vi "Talon Velocity Control.vi"(0 "CAN Talon SRX Ref":T1={"DeviceStatus"={"status"=FALSE, "code"=0, "source"=""}, "Type"=enum."PWM", "PWM"={"PWM Channel"=enum."PWM 1", "DeadBand"={"Name"="", "maxPositivePwm"=0, "minPositivePwm"=0, "centerPwm"=0, "maxNegativePwm"=0, "minNegativePwm"=0, "angularRange"=0}}, "CAN"={"Device Number"=0, "Control Mode"=enum."Percent VBus", "Semaphore"=refnum, "Max Vout"=12.0, "TalonSRX Control Mode"=enum."Percent VBus"}, "Invert"=FALSE}, 5 "PercentVoltage":dbl, 7 "Run to Speed?":bool, 9 "TargetSpeedRPM":dbl, 11 "error in (no error)":errorcluster) -> (4 "CAN Talon SRX Ref":T1={"DeviceStatus"={"status"=FALSE, "code"=0, "source"=""}, "Type"=enum."PWM", "PWM"={"PWM Channel"=enum."Invalid", "DeadBand"={"Name"="", "maxPositivePwm"=0, "minPositivePwm"=0, "centerPwm"=0, "maxNegativePwm"=0, "minNegativePwm"=0, "angularRange"=0}}, "CAN"={"Device Number"=0, "Control Mode"=enum."Percent VBus", "Semaphore"=refnum, "Max Vout"=12.0, "TalonSRX Control Mode"=enum."Percent VBus"}, "Invert"=FALSE}, 6 "Control Mode":T7, 10 "Motor Set":dbl, 15 "error out":errorcluster)   [LabVIEW 2015]
uses:
  <vilib>/Rock Robotics/WPI/MotorControl/WPI_MotorControlDeviceRef.ctl
  <vilib>/Rock Robotics/WPI/MotorControl/WPI_MotorControlType.ctl
  <vilib>/Rock Robotics/SystemInterfaces/DIO/FPGA_DIOPWMChannel.ctl
  <vilib>/Rock Robotics/WPI/PWM/WPI_PWMDeadband.ctl
  <vilib>/Rock Robotics/WPI/CAN/Jaguar/SubVIs/WPI_CANJaguar_ControlMode.ctl
  <vilib>/Rock Robotics/WPI/CAN/TalonSRX/WPI_CANTalonSRX_APIControlMode.ctl
  <vilib>/Rock Robotics/WPI/CAN/TalonSRX/WPI_CANTalonSRX_APIFeedbackSelect.ctl
panel:
  in  "PID stuff":T8
  out "SensorPosRotations":dbl
  out "Motor output Plot":cluster{"Applied Throttle":dbl}(graph)
  out "Target RPM":dbl
  out "SensorRPM Velocity RPM":dbl
  out "Applied Output":dbl
  out "Speed Closed Loop Plots":cluster{dbl, "Sensor Velocity":dbl}(graph)
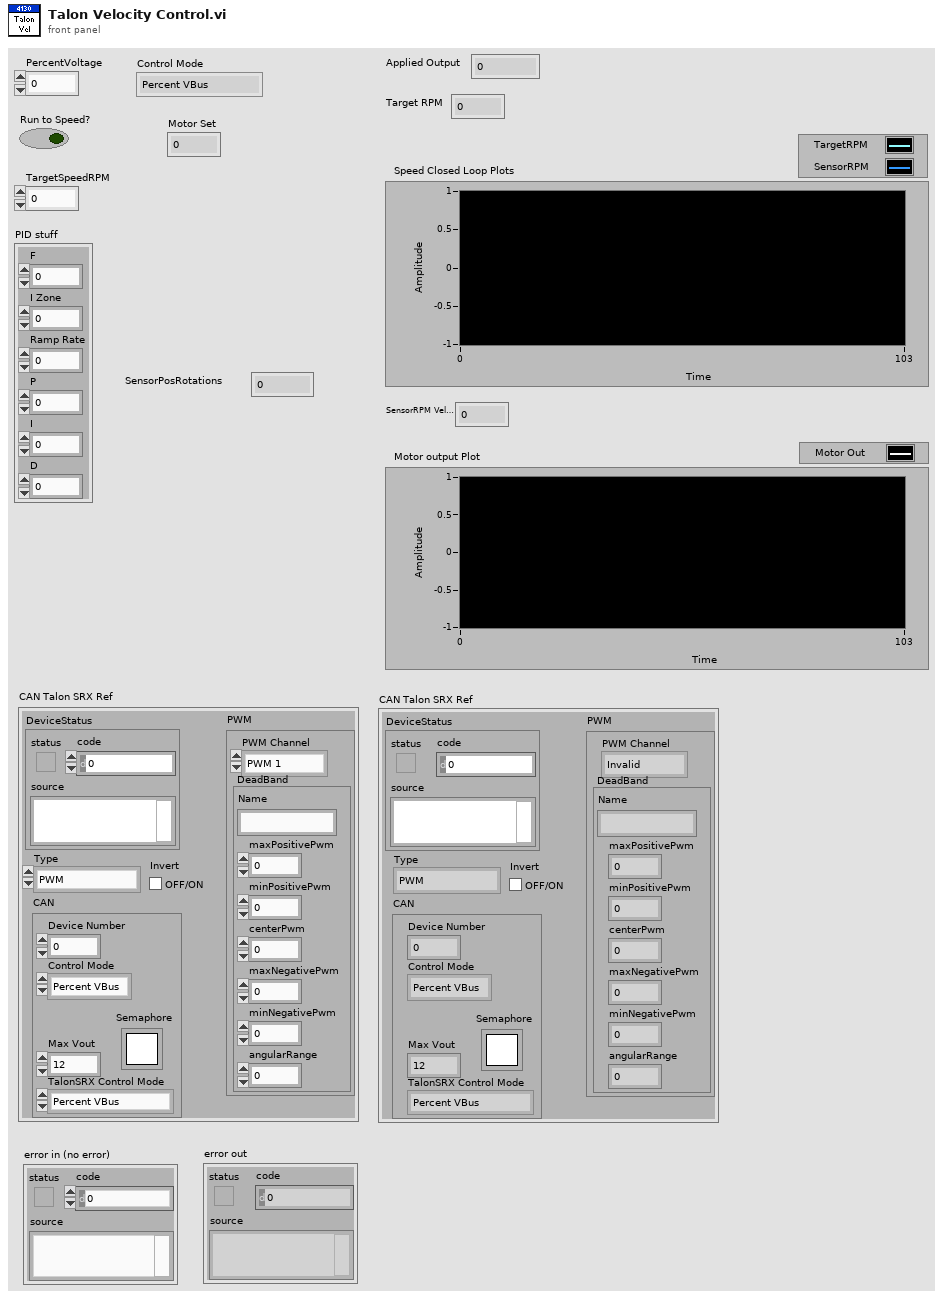
[diagram p1: front panel]
types:
  T1 = typedef "WPI_MotorControlDeviceRef.ctl" = cluster{"DeviceStatus":errorcluster, "Type":T2, "PWM":cluster{"PWM Channel":T3, "DeadBand":T4}, "CAN":cluster{"Device Number":u8, "Control Mode":T5, "Semaphore":T6, "Max Vout":dbl, "TalonSRX Control Mode":T7}, "Invert":bool}
  T2 = typedef "WPI_MotorControlType.ctl" = enum16{"PWM", "CAN", "CANTalonSRX"}
  T3 = typedef "FPGA_DIOPWMChannel.ctl" = enum8{"PWM 0", "PWM 1", "PWM 2", "PWM 3", "PWM 4", "PWM 5", "PWM 6", "PWM 7", "PWM 8", "PWM 9", "PWM MXP 0", "PWM MXP 1", "PWM MXP 2", "PWM MXP 3", "PWM MXP 4", "PWM MXP 5", "PWM MXP 6", "PWM MXP 7", "PWM MXP 8", "PWM MXP 9", "Invalid"}
  T4 = typedef "WPI_PWMDeadband.ctl" = cluster{"Name":string, "maxPositivePwm":i32, "minPositivePwm":i32, "centerPwm":i32, "maxNegativePwm":i32, "minNegativePwm":i32, "angularRange":u16}
  T5 = typedef "WPI_CANJaguar_ControlMode.ctl" = enum8{"Percent VBus", "Current", "Speed", "Position", "Voltage"}
  T6 = typedef "Semaphore RefNum" = refnum<k1>
  T7 = typedef "WPI_CANTalonSRX_APIControlMode.ctl" = enum8{"Percent VBus", "Speed", "Position", "Slave", "Unchanged / Invalid", "Voltage Compensation", "Current", "Motion Profile"}
  T8 = cluster{"F":dbl, "I Zone":dbl, "Ramp Rate":dbl, "P":dbl, "I":dbl, "D":dbl}
  T9 = typedef "WPI_CANTalonSRX_APIFeedbackSelect.ctl" = enum16{"Digital Quadrature Encoder", "Analog Potentiometer", "Analog Encoder", "Count on Quad-A (Rising-Edge)", "Count on Quad-A (Falling-Edge)", "CTR Magnetic Enc (Absolute)", "CTR Magnetic Enc (Relative)", "Pulse Width"}
  T10 = typedef "WPI_CANTalonSRX_GlobalStatus.ctl" = cluster{"Applied Throttle":dbl, "Module Enabled":bool, "CAN Error":errorcluster, "Closed Loop Error":dbl, "Forward Limit Switch Closed":bool, "Reverse Limit Switch Closed":bool, "Sensor Position":dbl, "Sensor Velocity":dbl, "Current":dbl, "Sticky Fault - Over Temp":bool, "Sticky Fault - Under Voltage":bool, "Sticky Fault - Forward Limit":bool, "Sticky Fault - Reverse Limit":bool, "Sticky Fault - Forward Soft Limit":bool, "Sticky Fault - Reverse Soft Limit":bool, "Brake is Enabled":bool, "Encoder Position":dbl, "Encoder Velocity":dbl, "Encoder Index Count":dbl, "Encoder A Pin State":bool, "Encoder B Pin State":bool, "Encoder Index Pin State":bool, "Analog In":dbl, "Analog In Velocity":dbl, "Temperature (C)":dbl, "Battery Voltage":dbl, "Control 5 Is Supported":bool, "Current Profile Slot Select":dbl, "Pos Div 8":bool, "Vel Div 4":bool, "Pulse Width Position":i32, "Pulse Width Velocity":i32, "Pulse Width Rise To Rise (us)":i32, "Pulse Width Rise To Fall (us)":i32, "Mot Prof Active Is Under Run":bool, "Mot Prof Active Has Under Run":bool, "Mot Prof Active Is Last":bool, "Mot Prof Active Velocity Only":bool, "Mot Prof Active Is Valid":bool, "Mot Prof Buffer Is Full":bool, "Mot Prof Active Profile Slot Select":i32, "Mot Prof NextID":i32, "Mot Prof Count":i32, "Mot Prof Active Velocity":dbl, "Mot Prof Active Position":dbl, "Mot Prof Output Enable":i32}
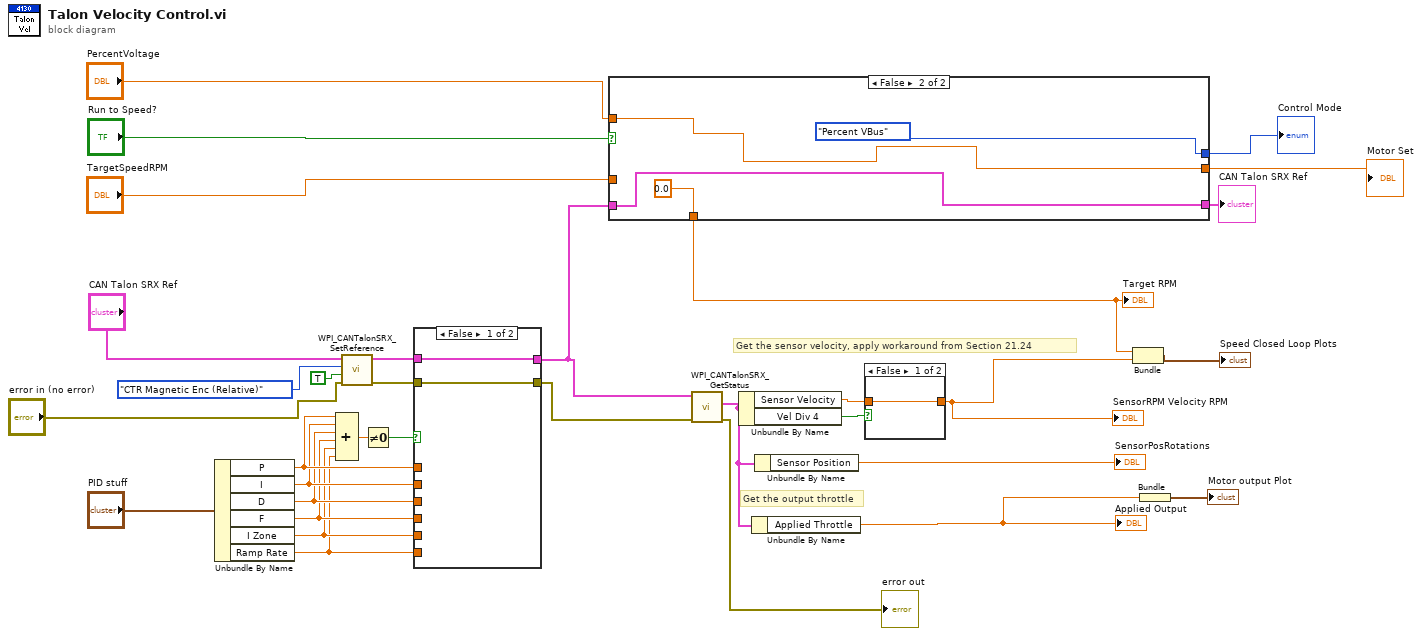
[diagram p0: block diagram]
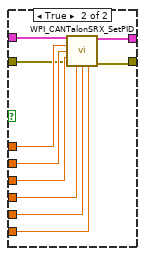
[diagram p2: hidden frame]
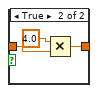
[diagram p3: hidden frame]
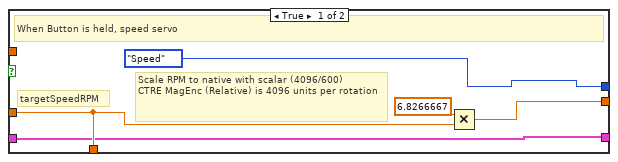
[diagram p4: hidden frame]
diagram:
  # "Get the output throttle"
  # "Get the sensor velocity, apply workaround from Section 21.24"
  n1 = Unbundle By Name("PID stuff") -> ("P"=w17:dbl, "I"=w16:dbl, "D"=w15:dbl, "F"=w14:dbl, "I Zone"=w13:dbl, "Ramp Rate"=w12:dbl)
  n2 = Compound Arithmetic op=ADD(w17, w16, w15, w14, w13, w12) -> (w11:dbl)
  n3 = call <vilib>:"WPI_CANTalonSRX_SetReference.vi"("error in (no error)"="error in (no error)", "Reverse Feedback Sensor"=TRUE, "Feedback Reference"=WPI_CANTalonSRX_APIFeedbackSelect."CTR Magnetic Enc (Relative)", "CAN Talon SRX Ref"="CAN Talon SRX Ref") -> ("error out"=w4:errorcluster, "CAN Talon SRX Ref"=w22:T1)  [unwired: 6 in]
  n4 = Not Equal To 0?(x=w11) -> (x != 0?=w10:bool)
  n5 = case shown="False" w10 {
    tunnel: [w35 w45] -> w26
    tunnel: w22 -> [w35 w44]
    tunnel: w17 -> [_ w43]
    tunnel: w16 -> [_ w42]
    tunnel: w15 -> [_ w41]
    tunnel: w14 -> [_ w40]
    tunnel: w13 -> [_ w39]
    tunnel: w12 -> [_ w38]
    tunnel: w4 -> [w34 w37]
    tunnel: [w34 w36] -> w3
    frame False {
    }
    frame True {
      n6 = call <vilib>:"WPI_CANTalonSRX_SetPID.vi"("CAN Talon SRX Ref"=w44, "P"=w43, "I"=w42, "D"=w41, "error in (no error)"=w37, "F"=w40, "I Zone"=w39, "Ramp Rate"=w38) -> ("CAN Talon SRX Ref"=w45:T1, "error out"=w36:errorcluster)  [unwired: 6 in]
    }
  }
  n7 = case shown="False" "Run to Speed?" {
    tunnel: "TargetSpeedRPM" -> [w49 _]
    tunnel: w26 -> [w47 w51]
    tunnel: [w49 0.0 ("x")] -> w29
    tunnel: "PercentVoltage" -> [_ w52]
    tunnel: [w48 w52] -> w8
    tunnel: [w47 w51] -> w7
    tunnel: [WPI_CANTalonSRX_APIControlMode."Speed" ("Control Mode") WPI_CANTalonSRX_APIControlMode."Percent VBus" ("Control Mode")] -> w9
    frame True {
      # "targetSpeedRPM"
      # "Scale RPM to native with scalar (4096/600)\nCTRE MagEnc (Relative) is 4096 units per rotation"
      # "When Button is held, speed servo"
      n8 = Multiply(x=6.8266667, y=w49) -> (x*y=w48:dbl)
    }
    frame False {
    }
  }
  "Target RPM" <- w29
  "Control Mode" <- w9
  "Motor Set" <- w8
  "CAN Talon SRX Ref" <- w7
  n9 = call <vilib>:"WPI_CANTalonSRX_GetStatus.vi"("error in (no error)"=w3, "CAN Talon SRX Ref"=w26) -> ("error out"=→"error out":errorcluster, "Talon SRX Status"=w24:T10)  [unwired: 7 in, 1 out]
  n10 = Unbundle By Name(w24) -> ("Sensor Velocity"=w19:dbl, "Vel Div 4"=w20:bool)
  n11 = Unbundle By Name(w24) -> ("Applied Throttle"=w28:dbl)
  "Applied Output" <- w28
  n12 = Unbundle By Name(w24) -> ("Sensor Position"=→"SensorPosRotations":dbl)
  n13 = case shown="False" w20 {
    tunnel: [w55 w57] -> w21
    tunnel: w19 -> [w55 w56]
    frame False {
    }
    frame True {
      n14 = Multiply(x=4.0, y=w56) -> (x*y=w57:dbl)
    }
  }
  "SensorRPM Velocity RPM" <- w21
  n15 = Bundle("x"=w29, "Sensor Velocity"=w21) -> (→"Speed Closed Loop Plots":cluster{"x":dbl, "Sensor Velocity":dbl})  [unwired: 1 in]
  n16 = Bundle("Applied Throttle"=w28) -> (→"Motor output Plot":cluster{"Applied Throttle":dbl})  [unwired: 1 in]
